vi "DMD_Control_PXI_Acq.vi"() -> ()   [LabVIEW 2016]
doc: "This example transfers a finite number of samples from the FPGA target to the Host using a stream."
uses:
  <vilib>/userdefined/Silver/nirio_resource_slv.ctl
  <vilib>/FPGAPlugInAG/PXIe-7961R/niLvFpga_Open_PXIe-7961R.vi
  <vilib>/rvi/interface/common/dynamic/niFpgaDynamicAddResources.vi
  <vilib>/FPGAPlugInAG/Dynamic/niLvFpga_Reset_Dynamic.vi
  <vilib>/FPGAPlugInAG/Dynamic/niLvFpga_Run_Dynamic.vi
  Library/error.llb/Error Cluster From Error Code.vi
  <vilib>/rvi/errors/niLvFpgaAdjustHostInterfaceError.vi
  <vilib>/FPGAPlugInAG/Dynamic/niLvFpga_Close_Dynamic.vi
  <vilib>/rvi/interface/nirviOpenFPGA/nirviOpenFPGA.xnode
  FPGA Bitfiles/DMDControlPXIAcq_PXIe-7961R_RIO7961R(FPGA)_hSkEQgsNMdM.lvbitx
  RIO 7961R (FPGA).vi
  <vilib>/rvi/interface/nirviMethod/nirviMethod.xnode
  <vilib>/rvi/interface/nirviCloseFPGA/nirviCloseFPGA.xnode
  <vilib>/FPGAPlugInAG/Dynamic/niLvFpga_WriteFifo_Dynamic.vi
  <vilib>/rvi/errors/niLvFpgaMergeErrorWithErrorCode.vi
panel:
  in  "Image Properties":T1={"Channel0 Properties"={"Basis 0"=0.0, "Swing 0"=2.931034482758621}, "Channel1 Properties"={"Basis 1"=0.0, "Swing 1"=2.931034482758621}, "Auto Swing"=FALSE} {"Channel1 Properties"."Swing 1" scale=0.0..5.0; "Channel1 Properties"."Basis 1" scale=0.0..0.5; "Channel0 Properties"."Basis 0" scale=0.0..0.5; "Channel0 Properties"."Swing 0" scale=0.0..5.0}
  in  "Parameters":T2={"RangeX"=30.0, "CentreY"=0.0, "CentreX"=38.0, "StepY"=3.0, "CentreZ"=0.0, "StepX"=3.0, "StepZ"=1.0, "RangeY"=30.0, "RangeZ"=1.0, "Z number"=0, "ZerM"=0.0, "ZerN"=0.0, "A"=0.0, "X number"=0, "Y number"=0}
  in  "Library Path":string
  out "Stripped Path":string
  out "aban num":u16
  out "fdiv num":u16
  in  "DMD Frequency":u32=20000 min=10 max=20000 format="%.0p"
  in  "PXI Clk":u32=80000000 format="%.0p"
  in  "New Window":bool
  out "Channel0":u32[][](array[numeric])
  out "Channel1":u32[][](array[numeric])
  out "RawData 1":dbl[](graph)
  out "ProjStartCont":i32
  in  "PictureTime/us":i32=48 min=0 max=256 step=1
  out "SeqAlloc":i32
  out "SequID":u32
  in  "Num of per rack":i32=200
  out "ErrorSeqPut":i32
  out "LoadingProgress":dbl(slide) scale=0.0..100.0
  out "DMD Type":string
  out "DeviceID":u32
  out "SerialNum":i32
  out "DevAlloc":i32
  out "Imaging":bool
  out "Projecting":bool
  out "Idle":bool
  out "Loading":bool
  out "No Patterns":bool
  out "PixelNum":i32=1
  in  "Stop":bool
  in  "Proj&Image":bool
  in  "Load patterns":bool
  in  "Free patterns":bool
  out "Raw Data 0":dbl[](graph)
  in  "Quit":bool
  out "Frame 1":T3(plugin-control)
  in  "Delay Time":u32(slide) scale=0.0..50.0
  out "Elements in Queue":i32
  in  "RIO Device":T4="RIO0"
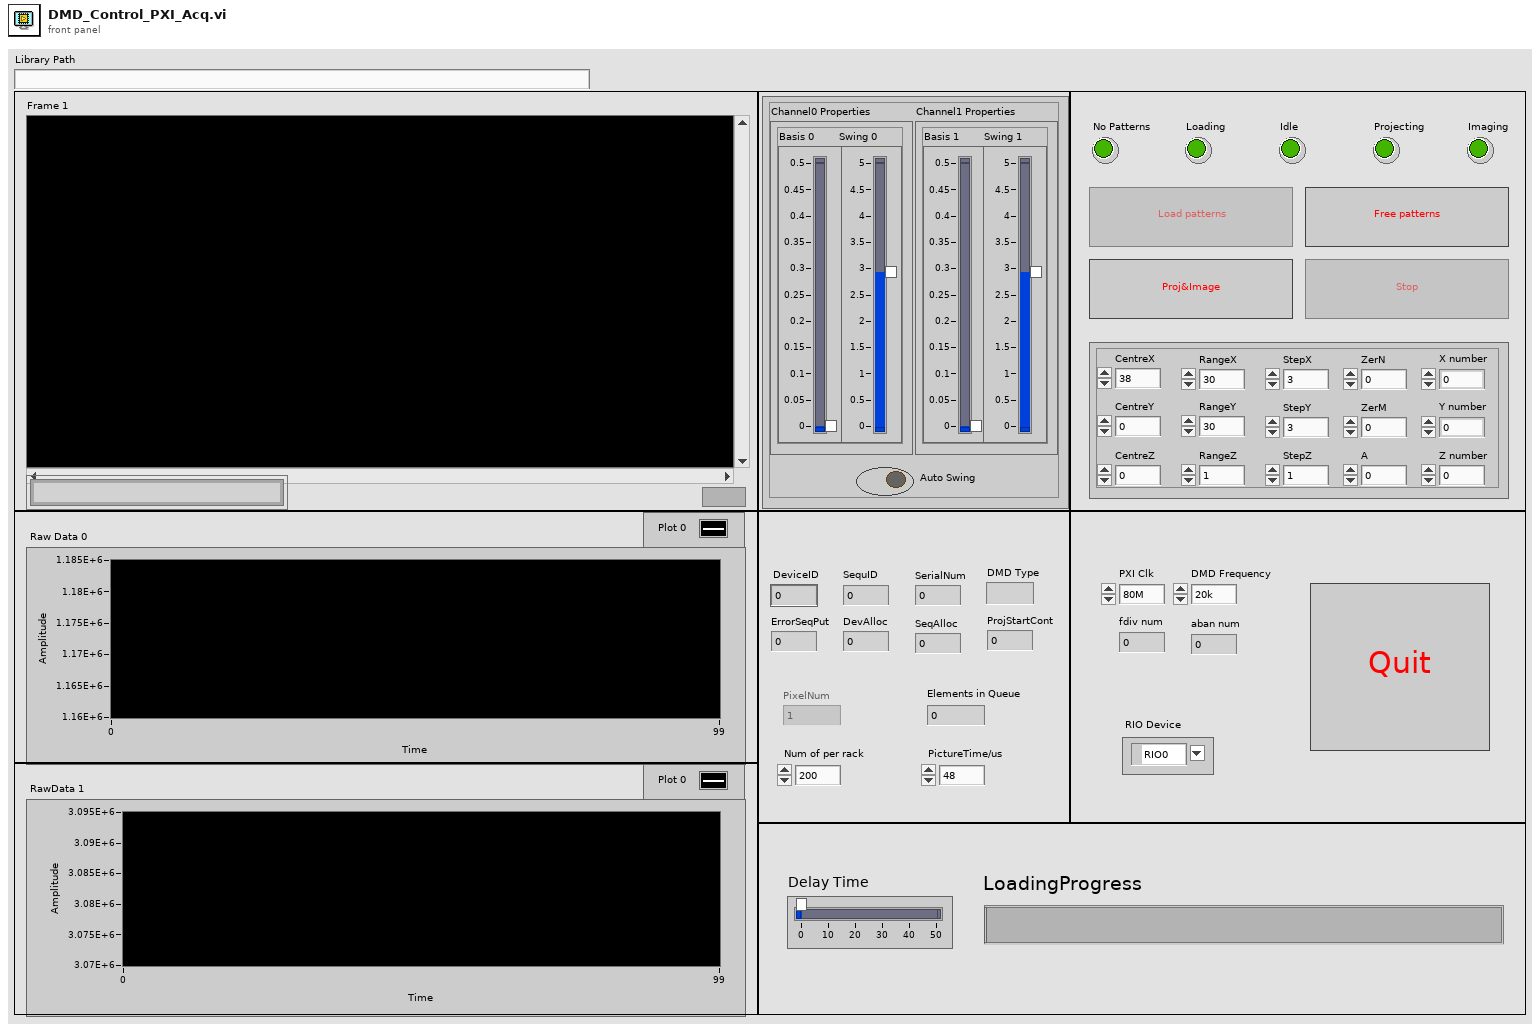
[diagram p1: front panel]
types:
  T1 = cluster{"Channel0 Properties":cluster{"Basis 0":dbl, "Swing 0":dbl}, "Channel1 Properties":cluster{"Basis 1":dbl, "Swing 1":dbl}, "Auto Swing":bool}
  T2 = cluster{"RangeX":dbl, "CentreY":dbl, "CentreX":dbl, "StepY":dbl, "CentreZ":dbl, "StepX":dbl, "StepZ":dbl, "RangeY":dbl, "RangeZ":dbl, "Z number":i32, "ZerM":dbl, "ZerN":dbl, "A":dbl, "X number":i32, "Y number":i32}
  T3 = typedef "IMAQ Image.ctl" = refnum<image>
  T4 = typedef "nirio_resource_slv.ctl" = tag
  T5 = enum8{"Enabled", "Disabled", "Disabled and Grayed Out"}
  T6 = enum16{"No sequence", "Load patterns", "Idle", "Project", "Imaging", "Free patterns"}
  T7 = enum32{"Invalid", "Standard", "Closed", "Hidden", "Minimized", "Maximized"}
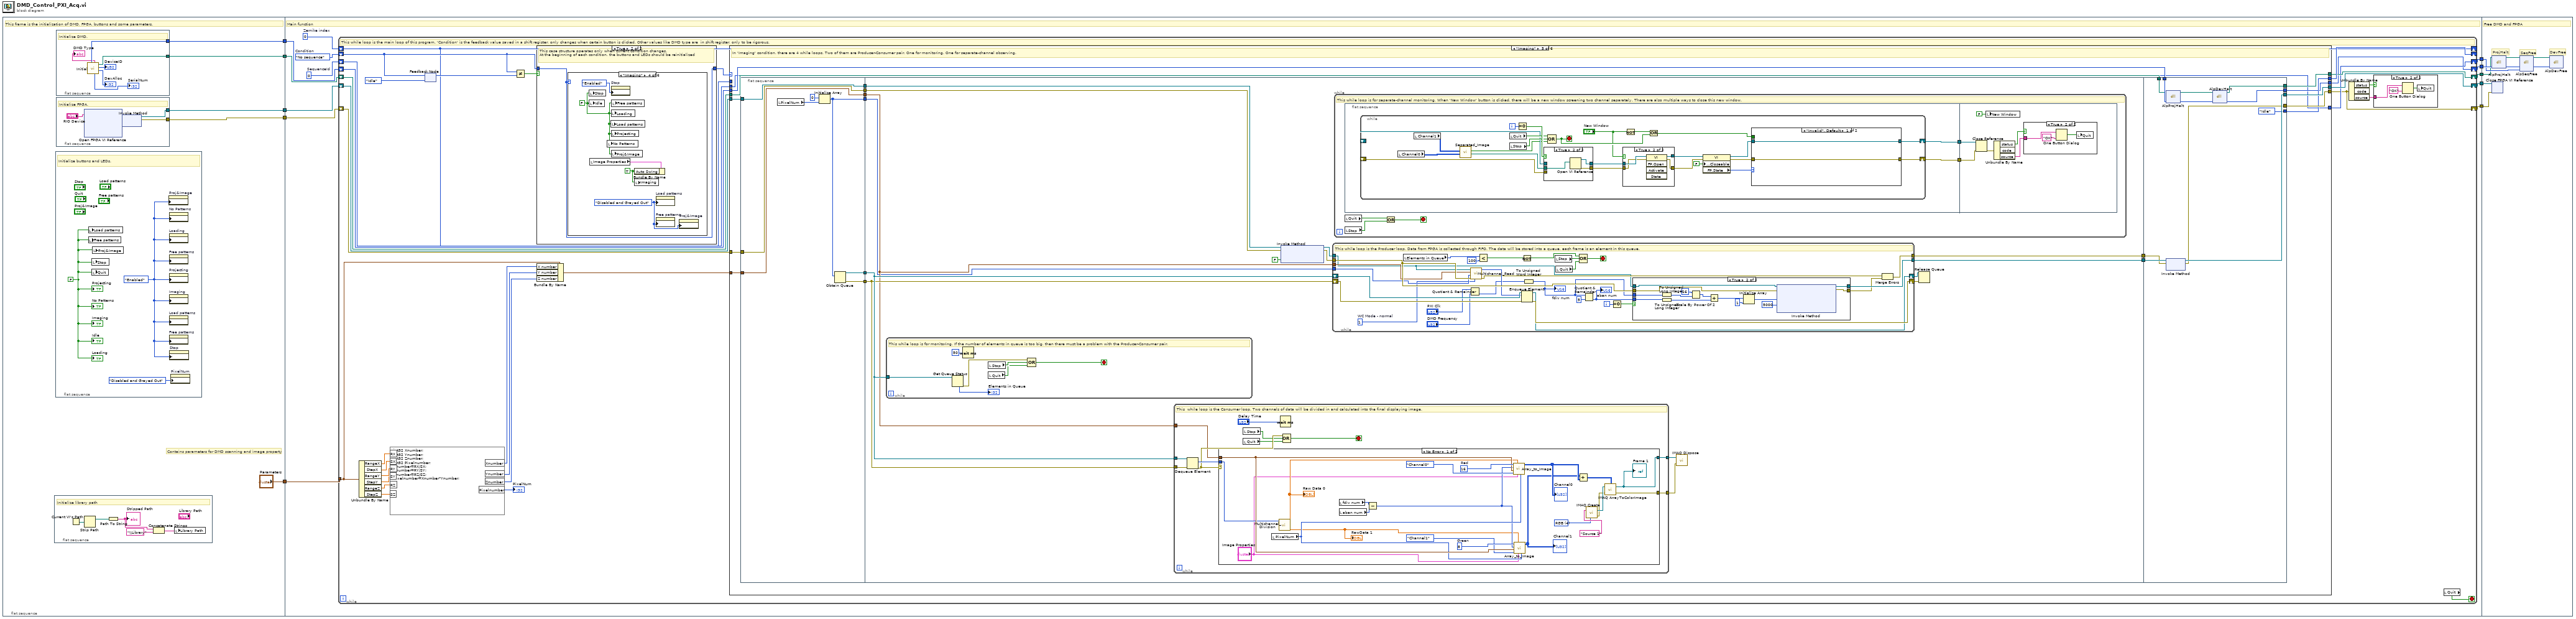
[diagram p0: block diagram]
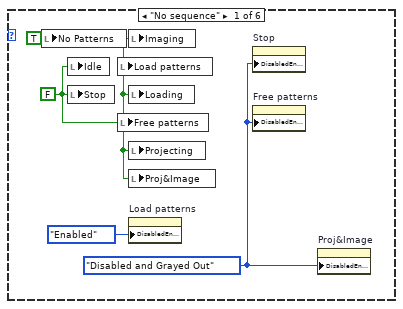
[diagram p4: hidden frame]
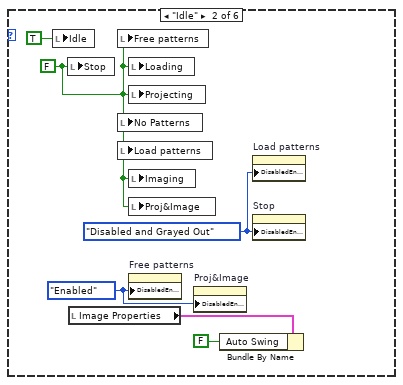
[diagram p5: hidden frame]
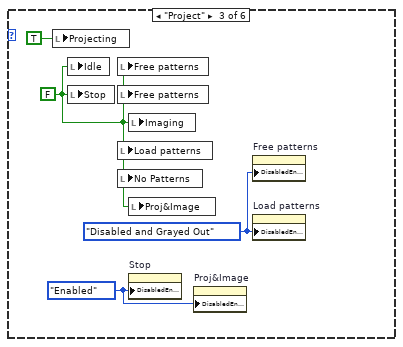
[diagram p6: hidden frame]
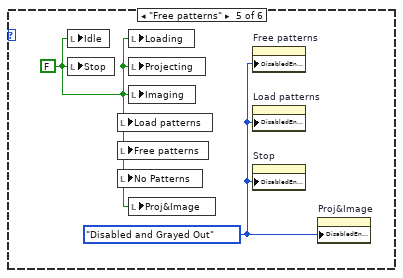
[diagram p7: hidden frame]
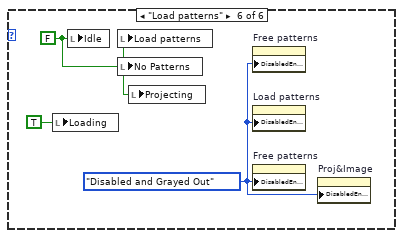
[diagram p8: hidden frame]
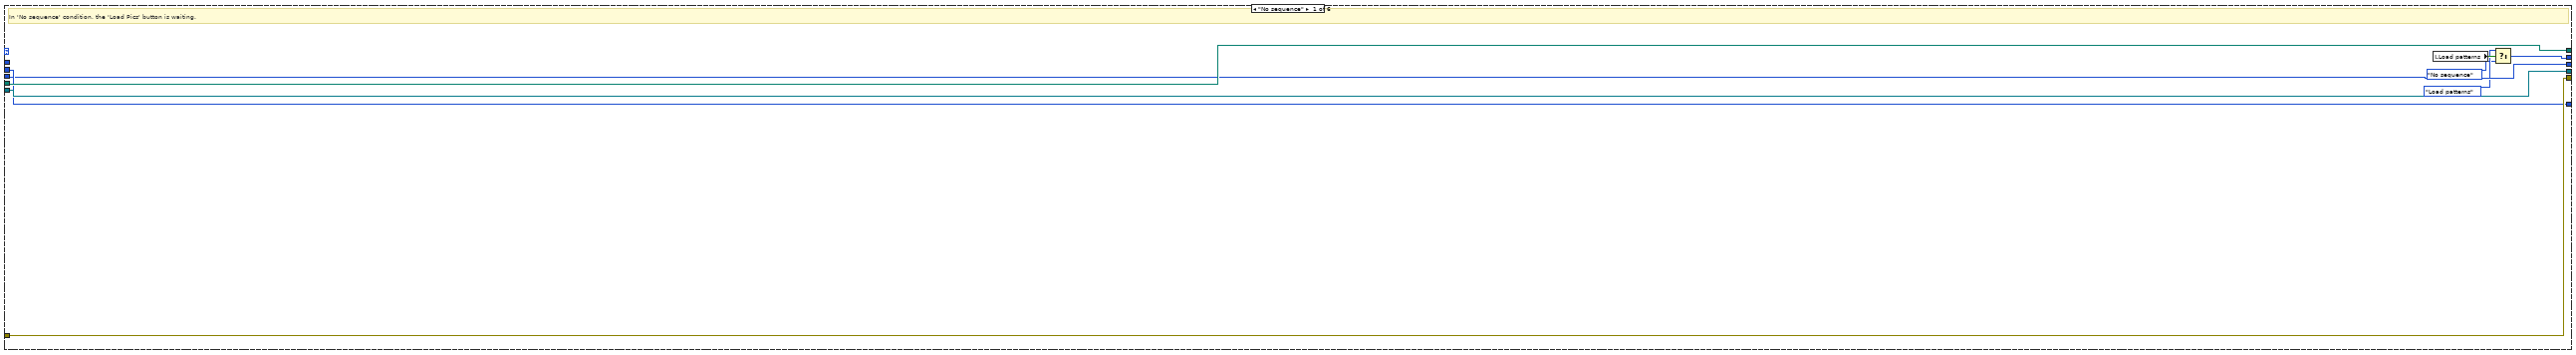
[diagram p9: hidden frame]
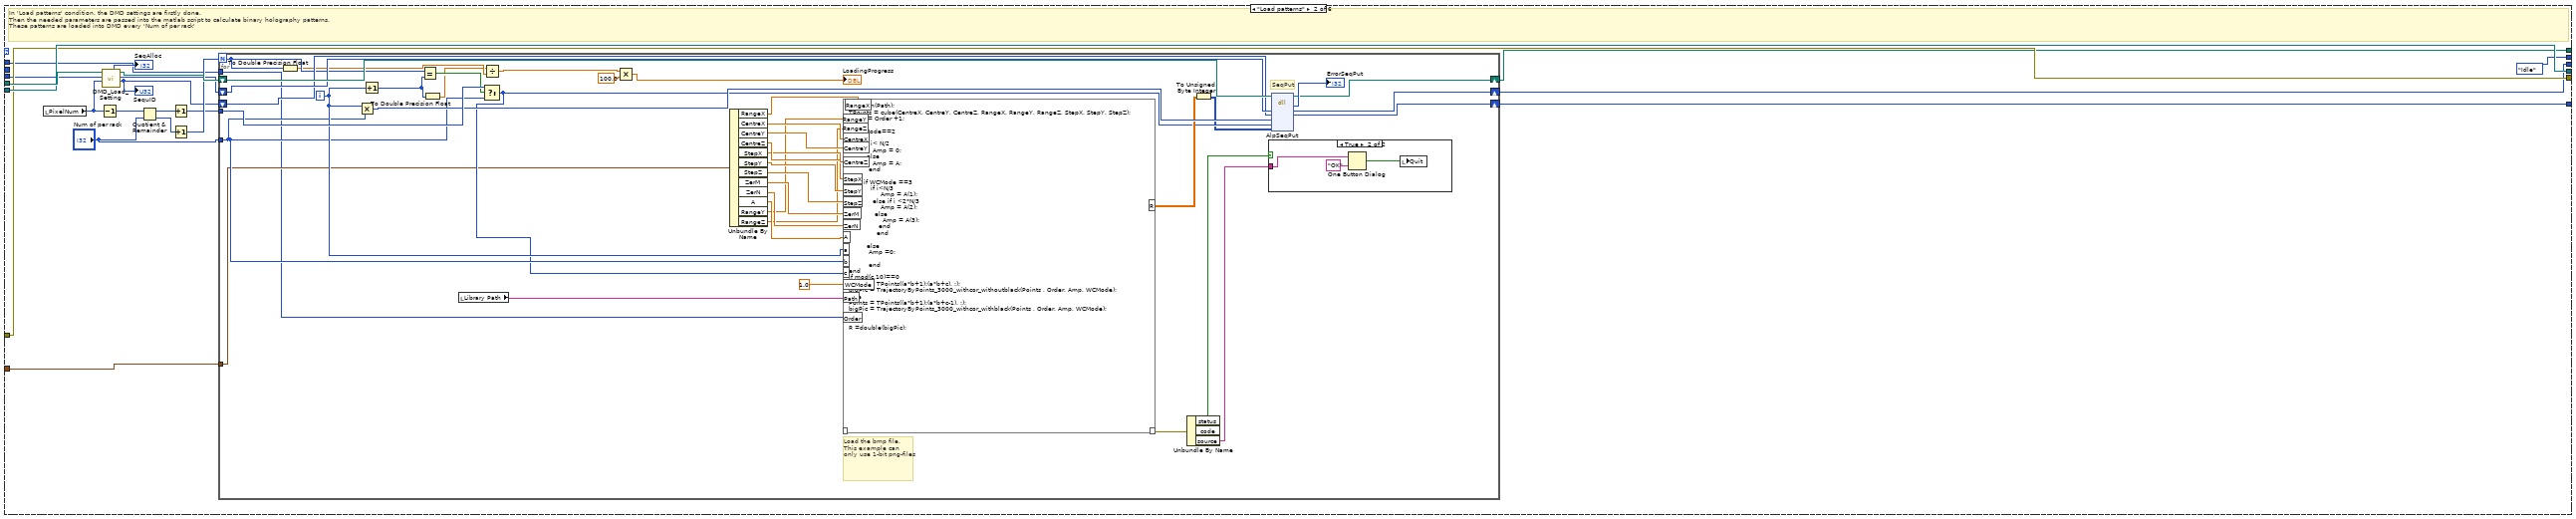
[diagram p10: hidden frame]
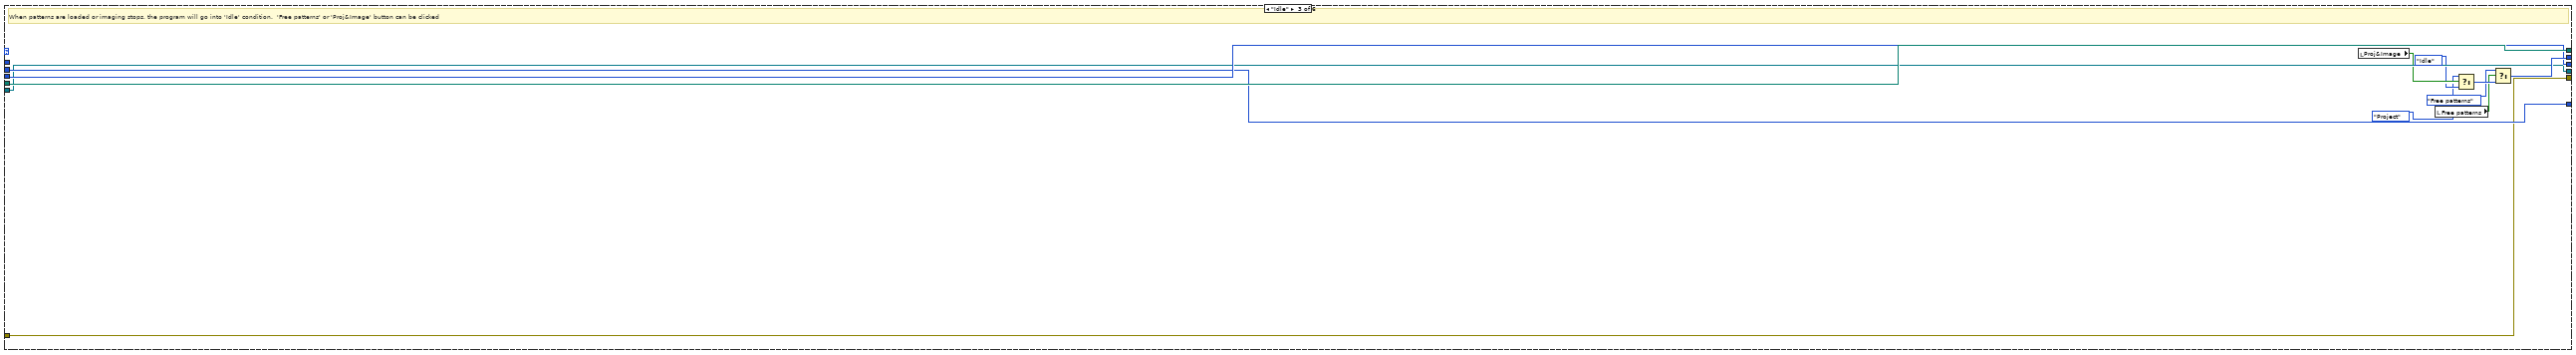
[diagram p12: hidden frame]
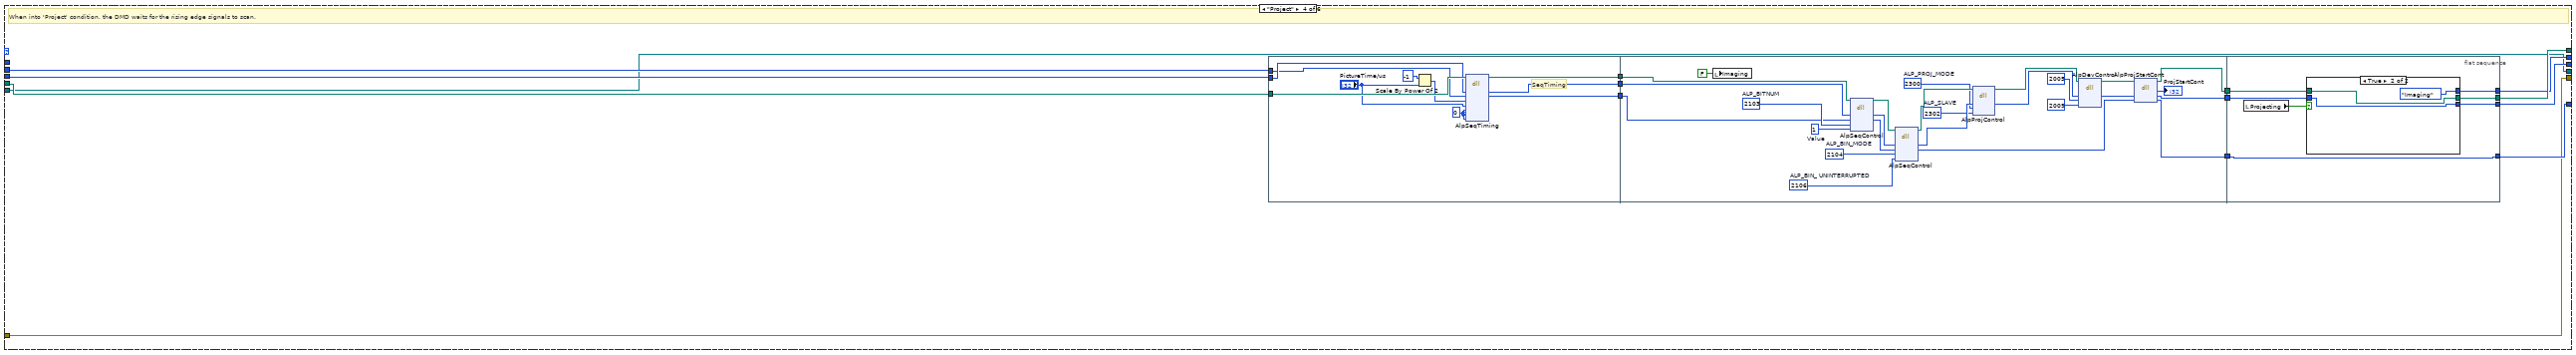
[diagram p13: hidden frame]
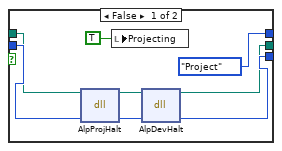
[diagram p14: hidden frame]
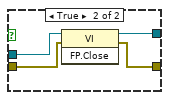
[diagram p16: hidden frame]
diagram:
  n1 = flat-sequence {
    tunnel: [w15] -> w10
    tunnel: [w14] -> w9
    tunnel: [w13] -> w8
    tunnel: [w12] -> w7
    tunnel: ["Parameters"] -> w1
    tunnel: w10 -> [w45]
    tunnel: w9 -> [w44]
    tunnel: w8 -> [w46]
    tunnel: w7 -> [w47]
    tunnel: [w42] -> w6
    tunnel: [w41] -> w5
    tunnel: [w40] -> w4
    tunnel: [w39] -> w3
    tunnel: [w38] -> w2
    tunnel: w1 -> [w36]
    tunnel: w6 -> [w483]
    tunnel: w5 -> [w482]
    tunnel: w4 -> [w481]
    tunnel: w3 -> [w480]
    tunnel: w2 -> [w479]
    frame #0 {
      # "Contains parameters for DMD scanning and image property"
      # "This frame is the initialization of DMD, FPGA, buttons and some parameters."
      n2 = flat-sequence {
        frame #0 {
          # "Initialize library path"
          n3 = Current VI's Path() -> (path=w18:path)
          n4 = Strip Path(path=w18) -> (stripped path=w17:path)  [unwired: 1 out]
          n5 = Path To String(path=w17) -> (string=w19:string)
          "Stripped Path" <- w19
          n6 = Concatenate Strings(w19, "\\Library" ("String")) -> (w16:string)
          n7 = local write "Library Path"(w16) -> ()
        }
      }
      n8 = flat-sequence {
        frame #0 {
          w32 = FALSE ("Idle")
          w34 = T5."Enabled" ("Disabled")
          # "Initialize buttons and LEDs."
          n9 = local write "Load patterns"(w32) -> ()
          n10 = local write "Free patterns"(w32) -> ()
          n11 = local write "Stop"(w32) -> ()
          n12 = local write "Quit"(w32) -> ()
          n13 = local write "Proj&Image"(w32) -> ()
          n14 = property on="Proj&Image" class="Bool (strict)"("DisabledEnum"=w34) -> ()  [unwired: 2 in, 2 out]
          n15 = property on="No Patterns" class="Bool (strict)"("DisabledEnum"=w34) -> ()  [unwired: 2 in, 2 out]
          n16 = property on="Loading" class="Bool (strict)"("DisabledEnum"=w34) -> ()  [unwired: 2 in, 2 out]
          n17 = property on="Free patterns" class="Bool (strict)"("DisabledEnum"=w34) -> ()  [unwired: 2 in, 2 out]
          n18 = property on="Projecting" class="Bool (strict)"("DisabledEnum"=w34) -> ()  [unwired: 2 in, 2 out]
          n19 = property on="Imaging" class="Bool (strict)"("DisabledEnum"=w34) -> ()  [unwired: 2 in, 2 out]
          n20 = property on="Load patterns" class="Bool (strict)"("DisabledEnum"=w34) -> ()  [unwired: 2 in, 2 out]
          n21 = property on="Free patterns" class="Bool (strict)"("DisabledEnum"=w34) -> ()  [unwired: 2 in, 2 out]
          n22 = property on="Stop" class="Bool (strict)"("DisabledEnum"=w34) -> ()  [unwired: 2 in, 2 out]
          n23 = property on="PixelNum" class="DigNum (strict)"("DisabledEnum"=T5."Disabled and Grayed Out" ("Disabled")) -> ()  [unwired: 2 in, 2 out]
          "Idle" <- w32
          "Imaging" <- w32
          "No Patterns" <- w32
          "Loading" <- w32
          "Projecting" <- w32
        }
      }
      n24 = flat-sequence {
        tunnel: [w29] -> w15
        tunnel: [w27] -> w12
        frame #0 {
          # "Initialize DMD."
          n25 = call "Initial.vi"() -> ("DevAlloc"=→"DevAlloc":i32, "DeviceID"=→"DeviceID":u32, "path out"=w29:path, "SerialNumber"=→"SerialNum":i32, "DMD Type"=→"DMD Type":string, "DeviceIdPtr"=w27:u32)  [unwired: 5 in, 1 out]
        }
      }
      n26 = flat-sequence {
        tunnel: [w25] -> w14
        tunnel: [w24] -> w13
        frame #0 {
          # "Initialize FPGA."
          n27 = xnode "Open FPGA VI Reference"("resource name"="RIO Device") -> ("FPGA VI Reference Out"=w22:refnum<k20>, "error out"=w21:errorcluster)  [unwired: 1 in]
          n28 = xnode "Invoke Method"("FPGA VI Reference In"=w22, "error in"=w21) -> ("FPGA VI Reference Out"=w25:refnum<k20>, "error out"=w24:errorcluster)
        }
      }
    }
    frame #1 {
      w35 = 0  # Zernike index
      w43 = u32 0  # SequenceId
      w37 = T6."No sequence"  # Condition
      # "Main function"
      n29 = while {
        shift-right: [w79] -> w42
        shift-left: w44 -> [w78]
        shift-right: [w52] -> w41
        shift-left: w46 -> [w77]
        shift-right: [w76] -> _
        shift-left: w37 -> [w67]
        shift-right: [w75] -> w38
        shift-left: w45 -> [w73]
        shift-right: [w74] -> w39
        shift-left: w43 -> [w72]
        shift-right: [w71] -> w40
        shift-left: w47 -> [w70]
        tunnel: w36 -> [w66]
        shift-right: [w48] -> _
        shift-left: w35 -> [w48]
        stop <- w53 stop-if-true
        # "This while loop is the main loop of this program. 'Condition' is the feedback value saved in a shift register, only changes when certain button is clicked. Other values like DMD type are  in shift register, only to be rigorous."
        n30 = Unbundle By Name(w66) -> ("RangeX"=w65:dbl, "StepX"=w64:dbl, "RangeY"=w63:dbl, "StepY"=w62:dbl, "RangeZ"=w61:dbl, "StepZ"=w60:dbl)
        n31 = formula code="int32 Xnumber;\nint32 Ynumber;\nint32 Znumber;\nint32 Pixelnumber;\nXnumber=RX/SX;\nYnumber=RY/SY;\nZnumber=RZ/SZ;\nPixelnumber=Xnumber*Ynumber;"("RX"=w65, "SX"=w64, "RY"=w63, "SY"=w62, "RZ"=w61, "SZ"=w60) -> ("Xnumber"=w59:i32, "Ynumber"=w58:i32, "Pixelnumber"=→"PixelNum":i32, "Znumber"=w56:i32)
        n32 = feedback-in #1(w67) -> ()
        n33 = feedback #1(T6."Idle") -> (w69:T6)
        n34 = Not Equal?(x=w67, y=w69) -> (x != y?=w68:bool)
        n35 = case shown="True" w68 {
          tunnel: w67 -> [w83 w84]
          tunnel: [w83 w84] -> w54
          frame False {
          }
          frame True {
            # "This case structure operates only when current condition changes.\nAt the beginning of each condition, the buttons and LEDs should be reinitialized"
            n36 = case shown="\"Imaging\"" w84 {
              frame "No sequence" {
                w85 = FALSE ("Idle")
                w86 = T5."Disabled and Grayed Out" ("Disabled")
                n37 = local write "No Patterns"(TRUE ("No pics")) -> ()
                n38 = local write "Idle"(w85) -> ()
                n39 = local write "Stop"(w85) -> ()
                n40 = local write "Load patterns"(w85) -> ()
                n41 = local write "Free patterns"(w85) -> ()
                n42 = local write "Imaging"(w85) -> ()
                n43 = local write "Loading"(w85) -> ()
                n44 = local write "Projecting"(w85) -> ()
                n45 = local write "Proj&Image"(w85) -> ()
                n46 = property on="Load patterns" class="Bool (strict)"("DisabledEnum"=T5."Enabled" ("Disabled")) -> ()  [unwired: 2 in, 2 out]
                n47 = property on="Stop" class="Bool (strict)"("DisabledEnum"=w86) -> ()  [unwired: 2 in, 2 out]
                n48 = property on="Free patterns" class="Bool (strict)"("DisabledEnum"=w86) -> ()  [unwired: 2 in, 2 out]
                n49 = property on="Proj&Image" class="Bool (strict)"("DisabledEnum"=w86) -> ()  [unwired: 2 in, 2 out]
              }
              frame "Idle" {
                w90 = T5."Enabled" ("Disabled")
                w93 = T5."Disabled and Grayed Out" ("Disabled")
                w91 = FALSE
                n50 = local write "Idle"(TRUE) -> ()
                n51 = local write "Stop"(w91) -> ()
                n52 = local read "Image Properties"() -> (w89:T1)
                n53 = local write "Free patterns"(w91) -> ()
                n54 = local write "No Patterns"(w91) -> ()
                n55 = local write "Load patterns"(w91) -> ()
                n56 = local write "Loading"(w91) -> ()
                n57 = local write "Projecting"(w91) -> ()
                n58 = local write "Imaging"(w91) -> ()
                n59 = local write "Proj&Image"(w91) -> ()
                n60 = property on="Free patterns" class="Bool (strict)"("DisabledEnum"=w90) -> ()  [unwired: 2 in, 2 out]
                n61 = property on="Proj&Image" class="Bool (strict)"("DisabledEnum"=w90) -> ()  [unwired: 2 in, 2 out]
                n62 = Bundle By Name(cluster=w89, "Auto Swing"=FALSE) -> ()  [unwired: 1 out]
                n63 = property on="Load patterns" class="Bool (strict)"("DisabledEnum"=w93) -> ()  [unwired: 2 in, 2 out]
                n64 = property on="Stop" class="Bool (strict)"("DisabledEnum"=w93) -> ()  [unwired: 2 in, 2 out]
              }
              frame "Project" {
                w98 = T5."Enabled" ("Disabled")
                w97 = T5."Disabled and Grayed Out" ("Disabled")
                w96 = FALSE
                n65 = local write "Projecting"(TRUE ("Projecting")) -> ()
                n66 = local write "Idle"(w96) -> ()
                n67 = local write "Stop"(w96) -> ()
                n68 = local write "Free patterns"(w96) -> ()
                n69 = local write "Free patterns"(w96) -> ()
                n70 = local write "Load patterns"(w96) -> ()
                n71 = local write "No Patterns"(w96) -> ()
                n72 = local write "Imaging"(w96) -> ()
                n73 = local write "Proj&Image"(w96) -> ()
                n74 = property on="Stop" class="Bool (strict)"("DisabledEnum"=w98) -> ()  [unwired: 2 in, 2 out]
                n75 = property on="Proj&Image" class="Bool (strict)"("DisabledEnum"=w98) -> ()  [unwired: 2 in, 2 out]
                n76 = property on="Free patterns" class="Bool (strict)"("DisabledEnum"=w97) -> ()  [unwired: 2 in, 2 out]
                n77 = property on="Load patterns" class="Bool (strict)"("DisabledEnum"=w97) -> ()  [unwired: 2 in, 2 out]
              }
              frame "Imaging" {
                w102 = T5."Disabled and Grayed Out" ("Disabled")
                w101 = TRUE
                w100 = FALSE
                n78 = local write "Stop"(w100) -> ()
                n79 = local write "Idle"(w100) -> ()
                n80 = local read "Image Properties"() -> (w99:T1)
                n81 = local write "No Patterns"(w100) -> ()
                n82 = local write "Load patterns"(w100) -> ()
                n83 = property on="Stop" class="Bool (strict)"("DisabledEnum"=T5."Enabled" ("Disabled")) -> ()  [unwired: 2 in, 2 out]
                n84 = local write "Loading"(w100) -> ()
                n85 = local write "Projecting"(w100) -> ()
                n86 = local write "Proj&Image"(w100) -> ()
                n87 = local write "Free patterns"(w100) -> ()
                n88 = Bundle By Name(cluster=w99, "Auto Swing"=w101) -> ()  [unwired: 1 out]
                n89 = local write "Imaging"(w101) -> ()
                n90 = property on="Load patterns" class="Bool (strict)"("DisabledEnum"=w102) -> ()  [unwired: 2 in, 2 out]
                n91 = property on="Free patterns" class="Bool (strict)"("DisabledEnum"=w102) -> ()  [unwired: 2 in, 2 out]
                n92 = property on="Proj&Image" class="Bool (strict)"("DisabledEnum"=w102) -> ()  [unwired: 2 in, 2 out]
              }
              frame "Free patterns" {
                w105 = T5."Disabled and Grayed Out" ("Disabled")
                w104 = FALSE
                n93 = local write "Idle"(w104) -> ()
                n94 = local write "Stop"(w104) -> ()
                n95 = local write "Load patterns"(w104) -> ()
                n96 = local write "Free patterns"(w104) -> ()
                n97 = local write "No Patterns"(w104) -> ()
                n98 = local write "Loading"(w104) -> ()
                n99 = local write "Projecting"(w104) -> ()
                n100 = local write "Imaging"(w104) -> ()
                n101 = local write "Proj&Image"(w104) -> ()
                n102 = property on="Free patterns" class="Bool (strict)"("DisabledEnum"=w105) -> ()  [unwired: 2 in, 2 out]
                n103 = property on="Load patterns" class="Bool (strict)"("DisabledEnum"=w105) -> ()  [unwired: 2 in, 2 out]
                n104 = property on="Stop" class="Bool (strict)"("DisabledEnum"=w105) -> ()  [unwired: 2 in, 2 out]
                n105 = property on="Proj&Image" class="Bool (strict)"("DisabledEnum"=w105) -> ()  [unwired: 2 in, 2 out]
              }
              frame "Load patterns" {
                w106 = T5."Disabled and Grayed Out" ("Disabled")
                w107 = FALSE
                n106 = local write "Loading"(TRUE) -> ()
                n107 = local write "Idle"(w107) -> ()
                n108 = local write "Load patterns"(w107) -> ()
                n109 = local write "No Patterns"(w107) -> ()
                n110 = local write "Projecting"(w107) -> ()
                n111 = property on="Free patterns" class="Bool (strict)"("DisabledEnum"=w106) -> ()  [unwired: 2 in, 2 out]
                n112 = property on="Load patterns" class="Bool (strict)"("DisabledEnum"=w106) -> ()  [unwired: 2 in, 2 out]
                n113 = property on="Free patterns" class="Bool (strict)"("DisabledEnum"=w106) -> ()  [unwired: 2 in, 2 out]
                n114 = property on="Proj&Image" class="Bool (strict)"("DisabledEnum"=w106) -> ()  [unwired: 2 in, 2 out]
              }
            }
          }
        }
        n115 = Bundle By Name(cluster=w66, "X number"=w59, "Y number"=w58, "Z number"=w56) -> (w55:T2)
        n116 = case shown="\"Imaging\"" w54 {
          tunnel: w78 -> [w117 w127 w188 w201 w278 w468]
          tunnel: w77 -> [w116 w126 w187 w203 w277 w467]
          tunnel: [w117 w127 w188 w201 w282 w468] -> w79
          tunnel: [w116 w126 w187 w203 w281 w467] -> w52
          tunnel: [w111 T6."Idle" w191 w202 w274 T6."No sequence"] -> w76
          tunnel: w70 -> [w112 w121 w190 w208 w273 w473]
          tunnel: w73 -> [w114 w130 w192 w209 w272 w474]
          tunnel: [w114 w125 w192 w206 w270 w471] -> w75
          tunnel: w72 -> [w113 _ w189 w207 w269 w472]
          tunnel: [w113 w128 w189 w205 w269 w469] -> w74
          tunnel: [w112 w124 w190 w204 w271 w470] -> w71
          tunnel: w55 -> [_ w122 _ _ w266 _]
          tunnel: w48 -> [_ w119 _ _ _ _]
          frame "No sequence" {
            # "In 'No sequence' condition, the 'Load Pics' button is waiting."
            n117 = local read "Load patterns"() -> (w115:bool)
            n118 = Select(t=T6."Load patterns", s=w115, f=T6."No sequence") -> (s? t:f=w111:T6)
          }
          frame "Load patterns" {
            # "In 'Load patterns' condition, the DMD settings are firstly done. \nThen the needed parameters are passed into the matlab script to calculate binary holography patterns. \nThese patterns are loaded into DMD every 'Num of per rack'"
            n119 = local read "PixelNum"() -> (w123:i32)
            n120 = Decrement(x=w123) -> (x-1=w136:i32)
            n121 = call "DMD_Load_Setting.vi"("PixelNum"=w123, "DeviceIdPtr"=w121, "path in"=w130) -> ("SequenceId"=w120:u32, "DeviceId"=w129:u32, "path out 2"=w137:path, "return type"=→"SeqAlloc":i32)  [unwired: 5 in]
            "SequID" <- w120
            n122 = Quotient & Remainder(x=w136, y="Num of per rack") -> (x-y*floor(x/y)=w133:i32, floor(x/y)=w138:i32)
            n123 = Increment(x=w133) -> (x+1=w132:i32)
            n124 = Increment(x=w138) -> (x+1=w134:i32)
            n125 = for {
              N: w134 -> [w161]
              shift-right: [w177] -> w125
              shift-left: w137 -> [w178]
              shift-right: [w175] -> w124
              shift-left: w129 -> [w176]
              shift-right: [w173] -> w128
              shift-left: w120 -> [w174]
              tunnel: "Num of per rack" -> [w164]
              tunnel: w132 -> [w172]
              tunnel: w122 -> [w157]
              tunnel: w119 -> [w139]
              i -> [w165]
              # "Load the bmp file.\nThis example can \nonly use 1-bit png-files"
              # "SeqPut"
              n126 = To Double Precision Float(number=w161) -> (double precision float=w160:dbl)
              n127 = Multiply(x=w165, y=w164) -> (x*y=w167:i32)
              n128 = Increment(x=w165) -> (x+1=w158:i32)
              n129 = Equal?(x=w161, y=w158) -> (x = y?=w171:bool)
              n130 = To Double Precision Float(number=w158) -> (double precision float=w159:dbl)
              n131 = local read "Library Path"() -> (w140:string)
              n132 = Select(t=w172, s=w171, f=w164) -> (s? t:f=w163:i32)
              n133 = Divide(x=w159, y=w160) -> (x/y=w170:dbl)
              n134 = Multiply(x=w170, y=100.0) -> (x*y=→"LoadingProgress":dbl)
              n135 = Unbundle By Name(w157) -> ("RangeX"=w156:dbl, "CentreX"=w155:dbl, "CentreY"=w154:dbl, "CentreZ"=w153:dbl, "StepX"=w152:dbl, "StepY"=w151:dbl, "StepZ"=w150:dbl, "ZerM"=w149:dbl, "ZerN"=w148:dbl, "A"=w147:dbl, "RangeY"=w146:dbl, "RangeZ"=w145:dbl)
              n136 = script code="addpath(Path);\nTPoints = cube(CentreX, CentreY, CentreZ, RangeX, RangeY, RangeZ, StepX, StepY, StepZ);\nOrder = Order +1;\n\nif WCMode==2\n     \n        if i< N/2\n            Amp = 0;\n         else\n            Amp = A;\n          end\n       \nelse if WCMode ==3\n           if i<N/3\n                Amp = A(1);\n            else if i <2*N/3\n                Amp = A(2);\n             else\n                 Amp = A(3);\n               end\n              end\n        \n         else \n          Amp =0;\n          \n          end\nend\nif mod(c,10)==0\nPoints = TPoints((a*b+1):(a*b+c), :);\nbigPic = TrajectoryByPoints_3000_withcor_withoutblack(Points , Order, Amp, WCMode);\nelse \nPoints = TPoints((a*b+1):(a*b+c-1), :);\nbigPic = TrajectoryByPoints_3000_withcor_withblack(Points , Order, Amp, WCMode);\nend\n\nR =double(bigPic);"("CentreX"=w155, "CentreY"=w154, "CentreZ"=w153, "StepX"=w152, "StepY"=w151, "StepZ"=w150, "ZerM"=w149, "ZerN"=w148, "A"=w147, "RangeX"=w156, "RangeY"=w146, "RangeZ"=w145, "a"=w165, "b"=w164, "c"=w163, "WCMode"=1.0 ("Real"), "Path"=w140, "Order"=w139) -> ("??"=w144:errorcluster, "R"=w166:dbl[][])  [unwired: 1 in]
              n137 = Unbundle By Name(w144) -> ("status"=w143:bool, "source"=w142:string)  [unwired: 1 out]
              n138 = To Unsigned Byte Integer(number=w166) -> (unsigned 8bit integer=w162:u8[][])
              n139 = case shown="True" w143 {
                tunnel: w142 -> [_ w182]
                frame False {
                }
                frame True {
                  n140 = One Button Dialog(message=w182, button name ("OK")="OK") -> (true=w180:bool)
                  n141 = local write "Quit"(w180) -> ()
                }
              }
              n142 = dll-call lib="?" fn="AlpSeqPut"(path in=w178, "DeviceId"=w176, "SequenceId"=w174, "PicOffset"=w167, "PicLoad"=w163, "UserArrayPtr"=w162) -> (path out=w177:path, "return type"=→"ErrorSeqPut":i32, "DeviceId"=w175:u32, "SequenceId"=w173:u32)  [unwired: 5 in, 1 out]
            }
          }
          frame "Idle" {
            # "When patterns are loaded or imaging stops, the program will go into 'Idle' condition.  'Free patterns' or 'Proj&Image' button can be clicked"
            n143 = local read "Proj&Image"() -> (w186:bool)
            n144 = local read "Free patterns"() -> (w193:bool)
            n145 = Select(t=T6."Project", s=w186, f=T6."Idle") -> (s? t:f=w194:T6)
            n146 = Select(t=T6."Free patterns", s=w193, f=w194) -> (s? t:f=w191:T6)
          }
          frame "Project" {
            # "When into 'Project' condition, the DMD waits for the rising edge signals to scan."
            n147 = flat-sequence {
              tunnel: w209 -> [w218]
              tunnel: [w217] -> w200
              tunnel: w208 -> [w216]
              tunnel: w207 -> [w215]
              tunnel: [w214] -> w199
              tunnel: [w213] -> w198
              tunnel: [w235] -> w197
              tunnel: w200 -> [w239]
              tunnel: w199 -> [w238]
              tunnel: w198 -> [w237]
              tunnel: [w236] -> w196
              tunnel: [w220] -> w195
              tunnel: w197 -> [w250]
              tunnel: [w252] -> w205
              tunnel: w196 -> [w252]
              tunnel: [w251] -> w202
              tunnel: [w249] -> w204
              tunnel: w195 -> [w248]
              tunnel: [w247] -> w206
              frame #0 {
                w219 = 0 ("element")
                # "SeqTiming"
                n148 = Scale By Power Of 2(n=i16 -1, x="PictureTime/us") -> (x*2^n=w210:i32)
                n149 = dll-call lib="C:/Users/CHEN Lab WorkStation/Desktop/LabVIEW Control Codes/alp4395.dll" fn="AlpSeqTiming"(path in=w218, "DeviceId"=w216, "SequenceId"=w215, "IlluminateTime"=w210, "PictureTime"="PictureTime/us", "TriggerDelay"=w219, "TriggerPulseWidth"=w219, "VdDelay"=w219) -> (path out=w217:path, "DeviceId"=w214:u32, "SequenceId"=w213:u32)  [unwired: 8 in, 1 out]
              }
              frame #1 {
                w231 = u32 2302  # ALP_SLAVE
                w232 = 2300  # ALP_PROJ_MODE
                w244 = 2106  # ALP_BIN_ UNINTERRUPTED
                w243 = 2104  # ALP_BIN_MODE
                w242 = 1  # Value
                w241 = 2103  # ALP_BITNUM
                n150 = local write "Imaging"(FALSE ("Project")) -> ()
                n151 = dll-call lib="C:/Users/CHEN Lab WorkStation/Desktop/LabVIEW Control Codes/alp4395.dll" fn="AlpSeqControl"(path in=w239, "DeviceId"=w238, "SequenceId"=w237, "ControlType"=w241, "ControlValue"=w242) -> (path out=w230:path, "DeviceId"=w229:u32, "SequenceId"=w228:u32)  [unwired: 5 in, 1 out]
                n152 = dll-call lib="C:/Users/CHEN Lab WorkStation/Desktop/LabVIEW Control Codes/alp4395.dll" fn="AlpSeqControl"(path in=w230, "DeviceId"=w229, "SequenceId"=w228, "ControlType"=w243, "ControlValue"=w244) -> (path out=w234:path, "DeviceId"=w233:u32, "SequenceId"=w227:u32)  [unwired: 5 in, 1 out]
                n153 = dll-call lib="C:/Users/CHEN Lab WorkStation/Desktop/LabVIEW Control Codes/alp4395.dll" fn="AlpProjControl"(path in=w234, "DeviceId"=w233, "ControlType"=w232, "ControlValue"=w231) -> (path out=w226:path, "DeviceId"=w224:u32)  [unwired: 5 in, 1 out]
                n154 = dll-call lib="C:/Users/CHEN Lab WorkStation/Desktop/LabVIEW Control Codes/alp4395.dll" fn="AlpDevControl"(path in=w226, "DeviceId"=w224, "ControlType"=2005, "ControlValue"=u32 2009) -> (path out=w225:path, "DeviceId"=w223:u32)  [unwired: 5 in, 1 out]
                n155 = dll-call lib="C:/Users/CHEN Lab WorkStation/Desktop/LabVIEW Control Codes/alp4395.dll" fn="AlpProjStartCont" ("alpD40.dll:AlpProjStart")(path in=w225, "DeviceId"=w223, "SequenceId"=w227) -> (path out=w220:path, "return type"=→"ProjStartCont":i32, "DeviceId"=w235:u32, "SequenceId"=w236:u32)  [unwired: 2 in, 1 out]
              }
              frame #2 {
                n156 = local read "Projecting"() -> (w246:bool)
                n157 = case shown="True" w246 {
                  tunnel: [T6."Project" T6."Imaging"] -> w251
                  tunnel: w250 -> [w260 w263]
                  tunnel: [w258 w263] -> w249
                  tunnel: w248 -> [w257 w262]
                  tunnel: [w255 w262] -> w247
                  frame False {
                    n158 = dll-call lib="C:/Users/CHEN Lab WorkStation/Desktop/summer_intern/Try5/alp4395.dll" fn="AlpProjHalt"(path in=w257, "DeviceId"=w260) -> (path out=w256:path, "DeviceId"=w259:u32)  [unwired: 3 in, 1 out]
                    n159 = local write "Projecting"(TRUE ("Projecting")) -> ()
                    n160 = dll-call lib="C:/Users/CHEN Lab WorkStation/Desktop/summer_intern/Try5/alp4395.dll" fn="AlpDevHalt" ("alpD40.dll:AlpProjHalt")(path in=w256, "DeviceId"=w259) -> (path out=w255:path, "DeviceId"=w258:u32)  [unwired: 3 in, 1 out]
                  }
                  frame True {
                  }
                }
              }
            }
          }
          frame "Imaging" {
            # "In 'Imaging' condition, there are 4 while loops. Two of them are Producer-Consumer pair. One for monitoring. One for separate-channel observing."
            n161 = flat-sequence {
              tunnel: w278 -> [w286]
              tunnel: w277 -> [w285]
              tunnel: [w286] -> w276
              tunnel: [w285] -> w275
              tunnel: [w289] -> w268
              tunnel: [w288] -> w267
              tunnel: w266 -> [w284]
              tunnel: [w284] -> w265
              tunnel: [w283] -> w264
              tunnel: [w305] -> w280
              tunnel: [w304] -> w279
              tunnel: w276 -> [w297]
              tunnel: w275 -> [w296]
              tunnel: w268 -> [w303]
              tunnel: w267 -> [w302]
              tunnel: w265 -> [w293]
              tunnel: w264 -> [w292]
              tunnel: [w462] -> w281
              tunnel: [w463] -> w282
              tunnel: w280 -> [w465]
              tunnel: w279 -> [w464]
              tunnel: [T6."Idle"] -> w274
              tunnel: w273 -> [w461]
              tunnel: w272 -> [w460]
              tunnel: [w459] -> w271
              tunnel: [w458] -> w270
              frame #0 {
                n162 = local read "PixelNum"() -> (w287:i32)
                n163 = Initialize Array(u64 0 ("element"), w287) -> (w283:u64[])
                n164 = Obtain Queue(element data type=w283) -> (queue out=w289:refnum<queue>, error out=w288:errorcluster)  [unwired: 4 in, 1 out]
              }
              frame #1 {
                n165 = while {
                  tunnel: w303 -> [w374]
                  stop <- w372 stop-if-true
                  # "This while loop is for monitoring. If the number of elements in queue is too big, then there must be a problem with the Producer-Consumer pair."
                  n166 = Get Queue Status(queue=w374) -> (error out=w373:errorcluster, # elements in queue=→"Elements in Queue":i32)  [unwired: 2 in, 6 out]
                  n167 = Wait (ms)(milliseconds to wait=u32 50) -> ()  [unwired: 1 out]
                  n168 = local read "Stop"() -> (w371:bool)
                  n169 = local read "Quit"() -> (w370:bool)
                  n170 = Compound Arithmetic op=OR(w373, w371, w370) -> (w372:bool)
                }
                n171 = while {
                  tunnel: w303 -> [w385]
                  tunnel: w302 -> [w384]
                  tunnel: [w383] -> w301
                  tunnel: [w382] -> w300
                  tunnel: w293 -> [w379]
                  stop <- w380 stop-if-true
                  # "This  while loop is the Consumer loop. Two channels of data will be divided in and calculated into the final displaying image."
                  n172 = Dequeue Element(queue=w385, error in (no error)=w384) -> (element=w386:u64[], error out=w381:errorcluster)  [unwired: 1 in, 2 out]
                  n173 = case shown="No Error" w381 {
                    tunnel: w386 -> [w391 _]
                    tunnel: [w409 _] -> w383
                    tunnel: [w408 _] -> w382
                    tunnel: w379 -> [w398 _]
                    frame No Error {
                      w399 = i16 8  # Green
                      w403 = i16 16  # Red
                      w404 = u32 4 items=["8 bits", "16 bits", "Float", "Complex", "RGB", "HSL"] ("Image Type")
                      n174 = local read "PixelNum"() -> (w396:i32)
                      n175 = call "Multichannel_Division.vi"("Array in"=w391) -> ("Array Out1"=w389:dbl[], "Array Out0"=w390:dbl[])  [unwired: 7 in]
                      "Raw Data 0" <- w390
                      "RawData 1" <- w389
                      n176 = local read "fdiv num"() -> (w394:u16)
                      n177 = local read "aban num"() -> (w393:u16)
                      n178 = Subtract(x=w394, y=w393) -> (x-y=w392:u16)
                      n179 = call "Array_to_Image.vi"("PixelNum"=w396, "Image Properties"="Image Properties", "Array"=w390, "Channel"=enum16{"Channel0", "Channel1"}."Channel0" ("Enum"), "Parameters"=w398, "Sum Num"=w392, "Color"=w403) -> ("Array"=w402:u32[][])  [unwired: 4 in]
                      "Channel0" <- w402
                      n180 = call "Array_to_Image.vi"("PixelNum"=w396, "Image Properties"="Image Properties", "Array"=w389, "Channel"=enum16{"Channel0", "Channel1"}."Channel1" ("Enum"), "Parameters"=w398, "Sum Num"=w392, "Color"=w399) -> ("Array"=w395:u32[][])  [unwired: 4 in]
                      "Channel1" <- w395
                      n181 = Add(x=w395, y=w402) -> (x+y=w401:u32[][])
                      n182 = call "IMAQ Create"("Image Name"="Source 1", "Image Type"=w404) -> ("New Image"=w406:T3, "error out"=w405:errorcluster)  [unwired: 3 in]
                      n183 = call "IMAQ ArrayToColorImage"("Image Pixels (U32)"=w401, "Image"=w406, "error in (no error)"=w405) -> ("Image Out"=w409:T3, "error out"=w408:errorcluster)  [unwired: 2 in]
                      "Frame 1" <- w409
                    }
                    frame Error {
                    }
                  }
                  n184 = local read "Stop"() -> (w378:bool)
                  n185 = local read "Quit"() -> (w377:bool)
                  n186 = Wait (ms)(milliseconds to wait="Delay Time") -> ()  [unwired: 1 out]
                  n187 = Compound Arithmetic op=OR(w381, w378, w377) -> (w380:bool)
                }
                n188 = xnode "Invoke Method"("FPGA VI Reference In"=w297, "error in"=w296, "Wait Until Done (F)"=FALSE) -> ("FPGA VI Reference Out"=w291:refnum<k20>, "error out"=w295:errorcluster)
                n189 = while {
                  tunnel: [w432] -> w305
                  tunnel: [w418] -> w304
                  shift-right: [w433] -> w299
                  shift-left: w303 -> [w438]
                  shift-right: [w434] -> w298
                  shift-left: w302 -> [w437]
                  tunnel: w291 -> [w411]
                  tunnel: w295 -> [w429]
                  tunnel: w292 -> [w428]
                  tunnel: w293 -> [w426]
                  i -> [w431]
                  stop <- w425 stop-if-true
                  w410 = 1  # WC Mode - normal
                  # "This while loop is the Producer loop. Data from FPGA is collected through FIFO. The data will be stored into a queue, each frame is an element in this queue."
                  n190 = local read "Elements in Queue"() -> (w436:i32)
                  n191 = Quotient & Remainder(x="PXI Clk", y="DMD Frequency") -> (floor(x/y)=w415:u32)  [unwired: 1 out]
                  n192 = call "Multichannel_Read.vi"("WC Mode"=w410, "error in (no error)"=w429, "Array in"=w428, "Cluster"=w426, "Refnum in"=w411) -> ("error out"=w420:errorcluster, "Array out"=w427:u64[])  [unwired: 5 in]
                  n193 = Less?(x=w436, y=100) -> (x < y?=w423:bool)
                  n194 = Not(x=w423) -> (.not. x?=w422:bool)
                  n195 = Enqueue Element(queue=w438, element=w427, error in (no error)=w437) -> (queue out=w433:refnum<queue>, error out=w434:errorcluster)  [unwired: 1 in, 1 out]
                  n196 = To Unsigned Word Integer(number=w415) -> (unsigned 16bit integer=w413:u16)
                  "fdiv num" <- w413
                  n197 = local read "Stop"() -> (w421:bool)
                  n198 = local read "Quit"() -> (w424:bool)
                  n199 = Compound Arithmetic op=OR(w422, w421, w424) -> (w425:bool)
                  n200 = Quotient & Remainder(x=w413, y=u16 5) -> (floor(x/y)=w412:u16)  [unwired: 1 out]
                  "aban num" <- w412
                  n201 = Equal To 0?(x=w431) -> (x = 0?=w430:bool)
                  n202 = case shown="True" w430 {
                    tunnel: [w440 w454] -> w432
                    tunnel: [w439 w453] -> w419
                    tunnel: w411 -> [w440 w452]
                    tunnel: w429 -> [w439 w451]
                    tunnel: w413 -> [_ w450]
                    tunnel: w412 -> [_ w449]
                    frame False {
                    }
                    frame True {
                      n203 = To Unsigned Long Integer(number=w450) -> (unsigned 32bit integer=w448:u32)
                      n204 = To Unsigned Long Integer(number=w449) -> (unsigned 32bit integer=w445:u32)
                      n205 = Scale By Power Of 2(n=i16 16, x=w448) -> (x*2^n=w446:u32)
                      n206 = Add(x=w446, y=w445) -> (x+y=w444:u32)
                      n207 = Initialize Array(w444, 1 ("dimension size")) -> (w442:u32[])
                      n208 = xnode "Invoke Method"("FPGA VI Reference In"=w452, "error in"=w451, "Data"=w442, "Timeout (ms)"=5000) -> ("FPGA VI Reference Out"=w454:refnum<k20>, "error out"=w453:errorcluster)  [unwired: 1 out]
                    }
                  }
                  n209 = Merge Errors(w420, w419) -> (w418:errorcluster)
                }
                n210 = while {
                  stop <- w306 stop-if-true
                  # "This while loop is for separate-channel monitoring, When 'New Window' button is clicked, there will be a new window screening two channel separately. There are also multiple ways to close this new window."
                  n211 = flat-sequence {
                    tunnel: [w312] -> w310
                    tunnel: [w311] -> w309
                    tunnel: w310 -> [w366]
                    tunnel: w309 -> [w365]
                    frame #0 {
                      n212 = while {
                        shift-right: [w320] -> w312
                        shift-left: _ -> [w319]
                        shift-right: [w315] -> w311
                        shift-left: _ -> [w314]
                        i -> [w336]
                        stop <- w325 stop-if-true
                        n213 = local read "Channel0"() -> (w334:u32[][])
                        n214 = local read "Channel1"() -> (w333:u32[][])
                        n215 = call "Separated_Image.vi"("Array"=w334, "Array 2"=w333) -> ("path"=w332:path, "stop 2"=w313:bool)  [unwired: 8 in]
                        n216 = local read "Quit"() -> (w327:bool)
                        n217 = local read "Stop"() -> (w326:bool)
                        n218 = Equal To 0?(x=w336) -> (x = 0?=w335:bool)
                        n219 = case shown="True" w335 {
                          tunnel: w332 -> [_ w360]
                          tunnel: [w357 w359] -> w331
                          tunnel: w319 -> [w357 _]
                          tunnel: [w356 w358] -> w318
                          tunnel: w314 -> [w356 _]
                          frame False {
                          }
                          frame True {
                            n220 = Open VI Reference(vi path=w360) -> (vi reference=w359:refnum<vi>, error out=w358:errorcluster)  [unwired: 5 in]
                          }
                        }
                        n221 = Compound Arithmetic op=OR(w327, w326, w313) -> (w325:bool)
                        n222 = case shown="True" "New Window" {
                          tunnel: w331 -> [w351 w355]
                          tunnel: [w351 w354] -> w330
                          tunnel: w318 -> [w350 w353]
                          tunnel: [w350 w352] -> w317
                          frame False {
                          }
                          frame True {
                            n223 = invoke class="VI" method="FP.Open"(reference=w355, error in=w353) -> (reference out=w354:refnum<vi>, error out=w352:errorcluster)  [unwired: 3 in, 3 out]
                          }
                        }
                        n224 = Not(x="New Window") -> (.not. x?=w321:bool)
                        n225 = Or(x=w321, y=w325) -> (x .or. y?=w324:bool)
                        n226 = property class="VI"(reference=w330, error in=w317, "Front Panel.Closeable"=FALSE ("Front Panel Window:Closeable")) -> (reference out=w323:refnum<vi>, error out=w316:errorcluster, "FP.State"=w328:T7)
                        n227 = case shown="\"Invalid\", Default" w328 {
                          tunnel: w324 -> [_ w343]
                          tunnel: w323 -> [w338 w342]
                          tunnel: [w338 w341] -> w320
                          tunnel: w316 -> [w337 w340]
                          tunnel: [w337 w339] -> w315
                          frame "Invalid", Default {
                          }
                          frame "Standard" {
                            n228 = case shown="False" w343 {
                              tunnel: w342 -> [w345 w349]
                              tunnel: [w345 w348] -> w341
                              tunnel: w340 -> [w344 w347]
                              tunnel: [w344 w346] -> w339
                              frame False {
                              }
                              frame True {
                                n229 = invoke class="VI" method="FP.Close"(reference=w349, error in=w347) -> (reference out=w348:refnum<vi>, error out=w346:errorcluster)  [unwired: 1 in, 1 out]
                              }
                            }
                          }
                        }
                      }
                    }
                    frame #1 {
                      n230 = Close Reference(reference=w366, error in (no error)=w365) -> (error out=w363:errorcluster)
                      n231 = local write "New Window"(FALSE ("New Window")) -> ()
                      n232 = Unbundle By Name(w363) -> ("status"=w362:bool, "source"=w361:string)  [unwired: 1 out]
                      n233 = case shown="True" w362 {
                        tunnel: w361 -> [_ w369]
                        frame False {
                        }
                        frame True {
                          n234 = One Button Dialog(message=w369, button name ("OK")="OK") -> (true=w367:bool)
                          n235 = local write "Quit"(w367) -> ()
                        }
                      }
                    }
                  }
                  n236 = local read "Quit"() -> (w307:bool)
                  n237 = local read "Stop"() -> (w308:bool)
                  n238 = Or(x=w307, y=w308) -> (x .or. y?=w306:bool)
                }
                n239 = call "IMAQ Dispose"("Image"=w301, "error in (no error)"=w300) -> ()  [unwired: 4 in, 1 out]
                n240 = Release Queue(queue=w299, error in (no error)=w298) -> ()  [unwired: 1 in, 3 out]
              }
              frame #2 {
                n241 = dll-call lib="D:/documents/Dropbox/Only me/wavefront_correction/LabVIEW Control Codes/LabVIEW Codes/alp4395.dll" fn="AlpProjHalt"(path in=w460, "DeviceId"=w461) -> (path out=w457:path, "DeviceId"=w456:u32)  [unwired: 3 in, 1 out]
                n242 = xnode "Invoke Method"("FPGA VI Reference In"=w465, "error in"=w464) -> ("FPGA VI Reference Out"=w463:refnum<k20>, "error out"=w462:errorcluster)
                n243 = dll-call lib="D:/documents/Dropbox/Only me/wavefront_correction/LabVIEW Control Codes/LabVIEW Codes/alp4395.dll" fn="AlpDevHalt"(path in=w457, "DeviceId"=w456) -> (path out=w458:path, "DeviceId"=w459:u32)  [unwired: 3 in, 1 out]
              }
            }
          }
          frame "Free patterns" {
            # "Free the patterns inside DMD."
            n244 = dll-call lib="?" fn="AlpSeqFree"(path in=w474, "DeviceId"=w473, "SequenceId"=w472) -> (path out=w471:path, "DeviceId"=w470:u32, "SequenceId"=w469:u32)  [unwired: 3 in, 1 out]
          }
        }
        n245 = Unbundle By Name(w52) -> ("status"=w50:bool, "source"=w51:string)  [unwired: 1 out]
        n246 = case shown="True" w50 {
          tunnel: w51 -> [_ w82]
          frame False {
          }
          frame True {
            n247 = One Button Dialog(message=w82, button name ("OK")="OK") -> (true=w80:bool)
            n248 = local write "Quit"(w80) -> ()
          }
        }
        n249 = local read "Quit"() -> (w53:bool)
      }
    }
    frame #2 {
      # "ProjHalt"
      # "SeqFree"
      # "DevFree"
      # "Free DMD and FPGA"
      n250 = dll-call lib="?" fn="AlpProjHalt"(path in=w479, "DeviceId"=w481) -> (path out=w475:path, "DeviceId"=w476:u32)  [unwired: 3 in, 1 out]
      n251 = xnode ("Close FPGA VI Reference")("FPGA VI Reference In"=w483, "error in"=w482) -> ()  [unwired: 1 out]
      n252 = dll-call lib="?" fn="AlpSeqFree"(path in=w475, "DeviceId"=w476, "SequenceId"=w480) -> (path out=w478:path, "DeviceId"=w477:u32)  [unwired: 4 in, 1 out]
      n253 = dll-call lib="?" fn="AlpDevFree"(path in=w478, "DeviceId"=w477) -> ()  [unwired: 4 in, 2 out]
    }
  }
